vi "1.3.7-UpdateDP.vi"(6 "allowed proximity squared":i16=400, 8 "Robot Y":i16, 9 "Robot X":i16, 10 "update lines or objects":enum16{"lines", "obstacles"}(ring)=enum."obstacles", 11 "Scan Number":u8) -> ()   [LabVIEW 2010]
uses:
  1.0-Hindbrain Global.vi
  Unsorted Files from Athena/behaviors/driveable path/drivable paths global.vi
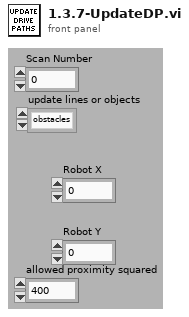
[diagram p1: front panel]
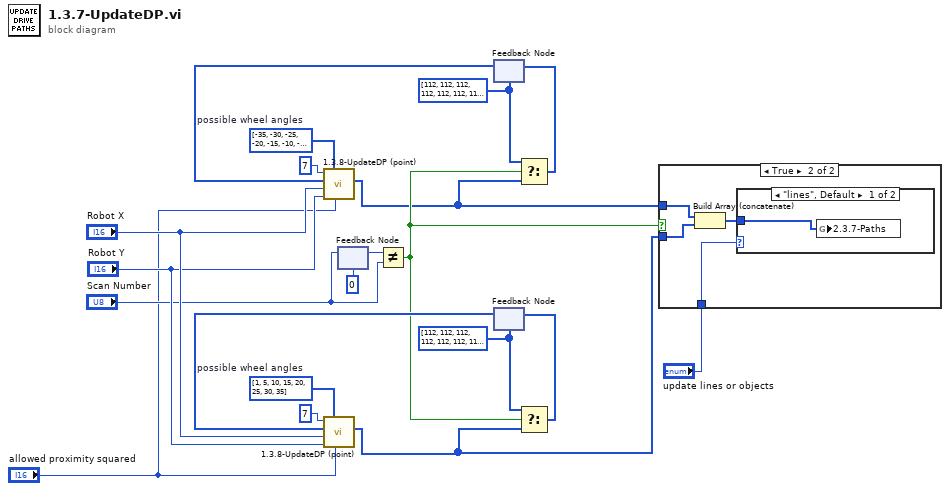
[diagram p0: block diagram]
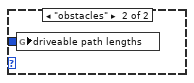
[diagram p3: hidden frame]
diagram:
  w9 = i8[] [1, 5, 10, 15, 20, 25, 30, 35]  # possible wheel angles
  w10 = i8[] [-35, -30, -25, -20, -15, -10, -5, -1]  # possible wheel angles
  w17 = u16[] [112, 112, 112, 112, 112, 112, 112, 112] ("updated max path lengths")
  w18 = u16[] [112, 112, 112, 112, 112, 112, 112, 112] ("updated max path lengths")
  n1 = feedback-in #1("Scan Number") -> ()
  n2 = feedback #1(u8 0 ("Scan Number")) -> (w7:u8)
  n3 = Not Equal?(x=w7, y="Scan Number") -> (x != y?=w5:bool)
  n4 = feedback #2(w18) -> (w19:u16[])
  n5 = call "1.3.8-UpdateDP (point).vi"("allowed proximity squared"="allowed proximity squared", "possible wheel angles"=w10, "y LIDAR position(in)"="Robot Y", "x LIDAR position(in)"="Robot X", "max path lengths"=w19, "number 16\" iterations"=7 ("number 16\" iterations")) -> ("updated max path lengths"=w3:u16[])  [unwired: 5 in]
  n6 = feedback #3(w17) -> (w16:u16[])
  n7 = call "1.3.8-UpdateDP (point).vi"("allowed proximity squared"="allowed proximity squared", "possible wheel angles"=w9, "y LIDAR position(in)"="Robot Y", "x LIDAR position(in)"="Robot X", "max path lengths"=w16, "number 16\" iterations"=7 ("number 16\" iterations")) -> ("updated max path lengths"=w14:u16[])  [unwired: 5 in]
  n8 = Select(t=w18, s=w5, f=w3) -> (s? t:f=w20:u16[])
  n9 = feedback-in #2(w20) -> ()
  n10 = Select(t=w17, s=w5, f=w14) -> (s? t:f=w15:u16[])
  n11 = feedback-in #3(w15) -> ()
  n12 = case shown="True" w5 {
    tunnel: w3 -> [_ w23]
    tunnel: w14 -> [_ w24]
    tunnel: "update lines or objects" -> [_ w21]
    frame False {
    }
    frame True {
      n13 = Build Array (concatenate)(w23, w24) -> (w22:u16[])
      n14 = case shown="\"lines\", Default" w21 {
        tunnel: w22 -> [w25 w26]
        frame "lines", Default {
          n15 = global write "1.0-Hindbrain Global.vi" "2.3.7-Paths"(w25) -> ()
        }
        frame "obstacles" {
          n16 = global write "drivable paths global.vi" "driveable path lengths"(w26) -> ()
        }
      }
    }
  }
